vi "create logbook.vi"   [LabVIEW 2018]
uses:
  Github/ICL-LabVIEW_General/Logbook/logbook states.ctl
  Github/ICL-LabVIEW_General/Logbook/logbook data.ctl
  <vilib>/Utility/sysdir.llb/System Directory Type.ctl
  Github/ICL-LabVIEW_General/Logbook/logbook library.lvlib
types:
  T1 = typedef "System Directory Type.ctl" = i32
  T2 = typedef "logbook data.ctl" = cluster{"path":path, "logbook ref":refnum<file>, "customHeader":string, "filename":string}
  T3 = typedef "logbook states.ctl" = enum16{"init", "open", "close", "new entry"}
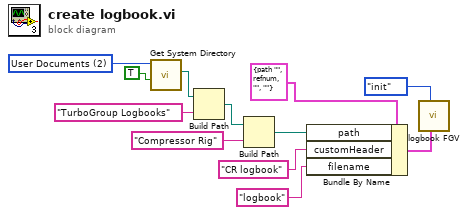
[diagram p0: block diagram]
diagram:
  w9 = T1 2 items=["User Home"=0, "User Desktop"=1, "User Documents"=2, "User Application Data"=3, "User Preferences"=4, "User Temporary"=5, "Public Documents"=6, "Public Application Data"=7, "Public Preferences"=8, "Public Cache"=13, "System Core Libraries"=9, "System Installed Libraries"=10, "Application Files"=11, "Boot Volume Root"=12] ("system directory type")
  n1 = call <vilib>:"Get System Directory.vi"("create directory if not found? (F)"=TRUE, "system directory type"=w9) -> ("system directory"=w7:path)  [unwired: 9 in]
  n2 = Build Path(base path=w7, name or relative path="TurboGroup Logbooks") -> (appended path=w5:path)
  n3 = Build Path(base path=w5, name or relative path="Compressor Rig") -> (appended path=w3:path)
  n4 = Bundle By Name(cluster=T2 {"path"=path "", "logbook ref"=refnum, "customHeader"="", "filename"=""}, "path"=w3, "customHeader"="CR logbook", "filename"="logbook") -> (w10:T2)
  n5 = call "logbook FGV.vi"(6:w10, "states"=logbook_states."init") -> ()  [unwired: 10 in]
